vi "Sagar C V Basic Gates Using NOR Gate.vi"() -> ()   [LabVIEW 2018]
panel:
  in  "?":string
  in  "?":string
  out "NOT GATE USING NOR GATE":bool
  out "OR GATE USING NOR GATE":bool
  out "AND GATE USING NOR GATE":bool
  in  "E":bool
  in  "D":bool
  in  "C":bool
  in  "B":bool
  in  "A":bool
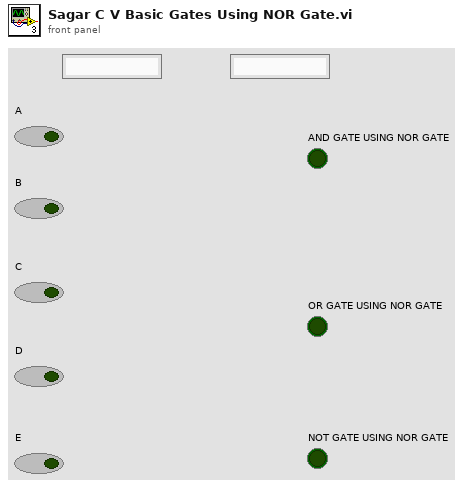
[diagram p1: front panel]
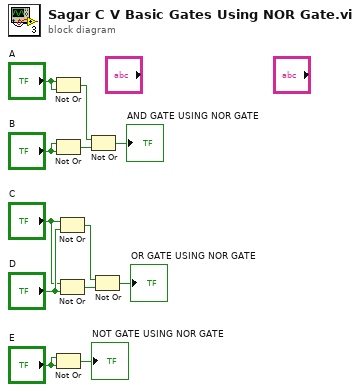
[diagram p0: block diagram]
diagram:
  n1 = Not Or(1:"A", 2:"A") -> (0:w10:bool)
  n2 = Not Or(1:"B", 2:"B") -> (0:w9:bool)
  n3 = Not Or(1:"E", 2:"E") -> (0:→"NOT GATE USING NOR GATE":bool)
  n4 = Not Or(1:"D", 2:"C") -> (0:w6:bool)
  n5 = Not Or(1:"D", 2:"C") -> (0:w5:bool)
  n6 = Not Or(1:w9, 2:w10) -> (0:→"AND GATE USING NOR GATE":bool)
  n7 = Not Or(1:w5, 2:w6) -> (0:→"OR GATE USING NOR GATE":bool)
